vi "Enable Secondary Display.vi"(8 "error in (no error)":errorcluster, 10 "Enable Secondary Display (T:Enable)":bool=TRUE, 11 "VISA resource name":refnum<visa-resource-name>) -> (0 "error out":errorcluster, 3 "VISA resource name out":refnum<visa-resource-name>)   [LabVIEW 2014, in "BK Precision 5491B.lvlib"]
doc: "Enables or disables the secondary display.\n\n<b>Note: Secondary display must be enabled first when reading both primary and secondary measurement readings using Read.vi</b>"
uses:
  <instrlib>/BK Precision 5491B/BK Precision 5491B.lvlib
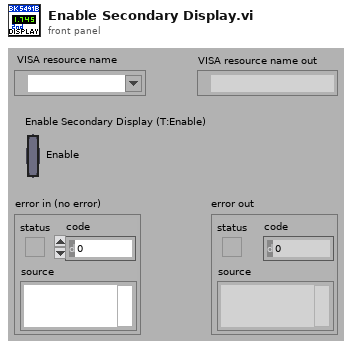
[diagram p1: front panel]
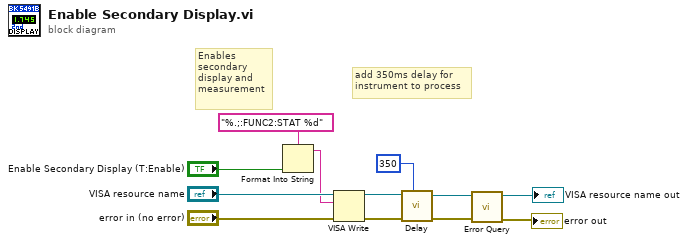
[diagram p0: block diagram]
diagram:
  # "add 350ms delay for\ninstrument to process"
  # "Enables\nsecondary\ndisplay and\nmeasurement"
  n1 = Format Into String(format string="%.;:FUNC2:STAT %d" ("write buffer"), "Enable Secondary Display (T:Enable)") -> (resulting string=w6:string)  [unwired: 2 in, 1 out]
  n2 = VISA Write(VISA resource name="VISA resource name", write buffer=w6, error in (no error)="error in (no error)") -> (VISA resource name out=w5:refnum<visa-resource-name>, error out=w4:errorcluster)  [unwired: 1 out]
  n3 = call <instrlib>:"Delay.vi"("Delay Time (0)"=u32 350, "error in (no error)"=w4, "VISA resource name"=w5) -> ("error out"=w3:errorcluster, "VISA resource name out"=w2:refnum<visa-resource-name>)  [unwired: 7 in]
  n4 = call <instrlib>:"Error Query.vi"("error in (no error)"=w3, "VISA resource name"=w2) -> ("error out"=→"error out":errorcluster, "VISA resource name out"=→"VISA resource name out":refnum<visa-resource-name>)  [unwired: 7 in, 1 out]
